vi "CloseIO.vi"   [LabVIEW 2012]
types:
  T1 = typedef "WPI_MotorControlDeviceRef.ctl" = cluster{"DeviceStatus":errorcluster, "Type":enum16{"PWM", "CAN"}, "PWM":cluster{"Digital Module":T2, "PWM Channel":T3, "DeadBand":T4}, "CAN":cluster{"Device Number":u8, "Control Mode":T5, "Semaphore":T6, "Max Vout":dbl}, "Invert":bool, "TransformRef":T7, "InvTransformRef":T7}
  T2 = typedef "FPGA_TypedefDigitalModule.ctl" = enum16{"Digital Module 1", "Digital Module 2"}
  T3 = typedef "FPGA_DIOPWMChannel.ctl" = enum8{"PWM 1", "PWM 2", "PWM 3", "PWM 4", "PWM 5", "PWM 6", "PWM 7", "PWM 8", "PWM 9", "PWM 10", "Invalid"}
  T4 = typedef "WPI_PWMDeadband.ctl" = cluster{"Name":string, "maxPositivePwm":i32, "minPositivePwm":i32, "centerPwm":i32, "maxNegativePwm":i32, "minNegativePwm":i32, "angularRange":u16}
  T5 = typedef "WPI_CANJaguar_ControlMode.ctl" = enum8{"Percent VBus", "Current", "Speed", "Position", "Voltage"}
  T6 = typedef "Semaphore RefNum" = refnum<k1>
  T7 = typedef "WPI_PWMTransform_ConPane.ctl" = refnum<vi>
  T8 = typedef "WPI_RobotDriveDevRef.ctl" = cluster{"DevStatus":errorcluster, "Motors[]":T1[], "Square Inputs":bool, "Max Output":dbl, "Isochronous":bool}
  T9 = typedef "WPI_DigitalInputDevRef.ctl" = cluster{"DevStatus":errorcluster, "DIO Channel":T10, "Digital Module":T2}
  T10 = typedef "FPGA_DIOChannel.ctl" = enum8{"DIO 1", "DIO 2", "DIO 3", "DIO 4", "DIO 5", "DIO 6", "DIO 7", "DIO 8", "DIO 9", "DIO 10", "DIO 11", "DIO 12", "DIO 13", "DIO 14", "Invalid"}
  T11 = typedef "WPI_CounterDevRef.ctl" = cluster{"DevStatus":errorcluster, "CntIndex":T12}
  T12 = typedef "FPGA_CounterCtrSystemIndex.ctl" = enum8{"Ctr 0", "Ctr 1", "Ctr 2", "Ctr 3", "Ctr 4", "Ctr 5", "Ctr 6", "Ctr 7", "Invalid"}
  T13 = typedef "WPI_EncoderDevRef.ctl" = cluster{"DevStatus":errorcluster, "EncoderIndex":T14, "CounterIndex":T12, "DistancePerCount":dbl, "Decoding Type":T15}
  T14 = typedef "FPGA_EncoderIdx.ctl" = enum8{"Enc 0", "Enc 1", "Enc 2", "Enc 3", "Invalid"}
  T15 = typedef "WPI_EncoderType.ctl" = enum16{"1x", "2x", "4x"}
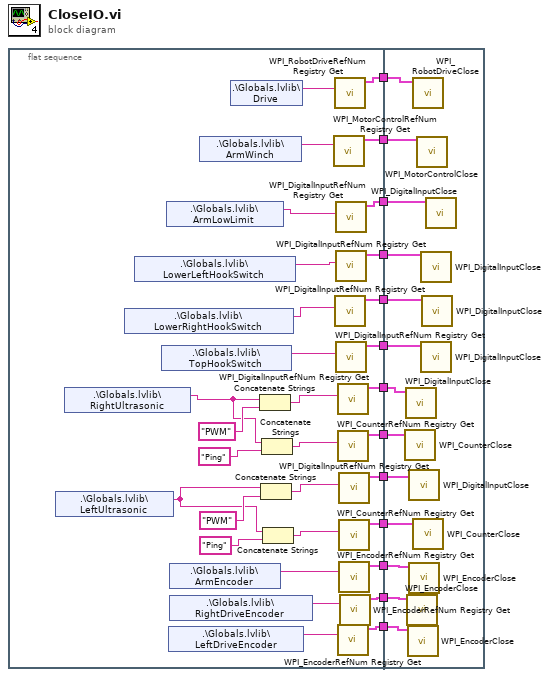
[diagram p0: block diagram]
diagram:
  n1 = flat-sequence {
    tunnel: [w43] -> w13
    tunnel: [w42] -> w12
    tunnel: [w27] -> w11
    tunnel: [w26] -> w10
    tunnel: [w25] -> w9
    tunnel: [w24] -> w8
    tunnel: [w23] -> w7
    tunnel: [w22] -> w6
    tunnel: [w21] -> w5
    tunnel: [w20] -> w4
    tunnel: [w18] -> w3
    tunnel: [w17] -> w2
    tunnel: [w14] -> w1
    tunnel: w13 -> [w58]
    tunnel: w12 -> [w57]
    tunnel: w11 -> [w56]
    tunnel: w10 -> [w55]
    tunnel: w9 -> [w54]
    tunnel: w8 -> [w53]
    tunnel: w7 -> [w52]
    tunnel: w6 -> [w51]
    tunnel: w5 -> [w50]
    tunnel: w4 -> [w49]
    tunnel: w3 -> [w48]
    tunnel: w2 -> [w47]
    tunnel: w1 -> [w46]
    frame #0 {
      n2 = shared-variable ".\\Globals.lvlib\\LeftUltrasonic"() -> (w29:string)  [unwired: 1 in, 1 out]
      n3 = shared-variable ".\\Globals.lvlib\\RightUltrasonic"() -> (w35:string)  [unwired: 1 in, 1 out]
      n4 = shared-variable ".\\Globals.lvlib\\LowerRightHookSwitch"() -> (w39:string)  [unwired: 1 in, 1 out]
      n5 = shared-variable ".\\Globals.lvlib\\LowerLeftHookSwitch"() -> (w40:string)  [unwired: 1 in, 1 out]
      n6 = shared-variable ".\\Globals.lvlib\\TopHookSwitch"() -> (w38:string)  [unwired: 1 in, 1 out]
      n7 = shared-variable ".\\Globals.lvlib\\ArmLowLimit"() -> (w41:string)  [unwired: 1 in, 1 out]
      n8 = shared-variable ".\\Globals.lvlib\\LeftDriveEncoder"() -> (w15:string)  [unwired: 1 in, 1 out]
      n9 = shared-variable ".\\Globals.lvlib\\ArmEncoder"() -> (w16:string)  [unwired: 1 in, 1 out]
      n10 = shared-variable ".\\Globals.lvlib\\RightDriveEncoder"() -> (w19:string)  [unwired: 1 in, 1 out]
      n11 = shared-variable ".\\Globals.lvlib\\ArmWinch"() -> (w44:string)  [unwired: 1 in, 1 out]
      n12 = shared-variable ".\\Globals.lvlib\\Drive"() -> (w45:string)  [unwired: 1 in, 1 out]
      n13 = Concatenate Strings(w35, "PWM") -> (w36:string)
      n14 = Concatenate Strings(w29, "PWM") -> (w31:string)
      n15 = Concatenate Strings(w35, "Ping") -> (w33:string)
      n16 = Concatenate Strings(w29, "Ping") -> (w32:string)
      n17 = call <vilib>:"WPI_MotorControlRefNum Registry Get.vi"("refnum name"=w44) -> ("MotorControlDevRef"=w42:T1)  [unwired: 9 in, 1 out]
      n18 = call <vilib>:"WPI_RobotDriveRefNum Registry Get.vi"("refnum name"=w45) -> ("RobotDriveDevRef"=w43:T8)  [unwired: 9 in, 1 out]
      n19 = call <vilib>:"WPI_DigitalInputRefNum Registry Get.vi"("refnum name"=w39) -> ("DigitalInputDevRef"=w24:T9)  [unwired: 9 in, 1 out]
      n20 = call <vilib>:"WPI_DigitalInputRefNum Registry Get.vi"("refnum name"=w41) -> ("DigitalInputDevRef"=w22:T9)  [unwired: 9 in, 1 out]
      n21 = call <vilib>:"WPI_DigitalInputRefNum Registry Get.vi"("refnum name"=w40) -> ("DigitalInputDevRef"=w23:T9)  [unwired: 9 in, 1 out]
      n22 = call <vilib>:"WPI_DigitalInputRefNum Registry Get.vi"("refnum name"=w38) -> ("DigitalInputDevRef"=w25:T9)  [unwired: 9 in, 1 out]
      n23 = call <vilib>:"WPI_DigitalInputRefNum Registry Get.vi"("refnum name"=w36) -> ("DigitalInputDevRef"=w26:T9)  [unwired: 9 in, 1 out]
      n24 = call <vilib>:"WPI_CounterRefNum Registry Get.vi"("refnum name"=w33) -> ("CounterDevRef"=w20:T11)  [unwired: 9 in, 1 out]
      n25 = call <vilib>:"WPI_EncoderRefNum Registry Get.vi"("refnum name"=w15) -> ("EncoderDevRef"=w14:T13)  [unwired: 9 in, 1 out]
      n26 = call <vilib>:"WPI_DigitalInputRefNum Registry Get.vi"("refnum name"=w31) -> ("DigitalInputDevRef"=w27:T9)  [unwired: 9 in, 1 out]
      n27 = call <vilib>:"WPI_CounterRefNum Registry Get.vi"("refnum name"=w32) -> ("CounterDevRef"=w21:T11)  [unwired: 9 in, 1 out]
      n28 = call <vilib>:"WPI_EncoderRefNum Registry Get.vi"("refnum name"=w16) -> ("EncoderDevRef"=w17:T13)  [unwired: 9 in, 1 out]
      n29 = call <vilib>:"WPI_EncoderRefNum Registry Get.vi"("refnum name"=w19) -> ("EncoderDevRef"=w18:T13)  [unwired: 9 in, 1 out]
    }
    frame #1 {
      n30 = call <vilib>:"WPI_CounterClose.vi"("CounterDevRef"=w49) -> ()  [unwired: 10 in, 1 out]
      n31 = call <vilib>:"WPI_DigitalInputClose.vi"("DigitalInputDevRef"=w55) -> ()  [unwired: 10 in, 1 out]
      n32 = call <vilib>:"WPI_EncoderClose.vi"("EncoderDevRef"=w48) -> ()  [unwired: 10 in, 1 out]
      n33 = call <vilib>:"WPI_EncoderClose.vi"("EncoderDevRef"=w46) -> ()  [unwired: 10 in, 1 out]
      n34 = call <vilib>:"WPI_DigitalInputClose.vi"("DigitalInputDevRef"=w56) -> ()  [unwired: 10 in, 1 out]
      n35 = call <vilib>:"WPI_EncoderClose.vi"("EncoderDevRef"=w47) -> ()  [unwired: 10 in, 1 out]
      n36 = call <vilib>:"WPI_RobotDriveClose.vi"("RobotDriveDevRef"=w58) -> ()  [unwired: 10 in, 1 out]
      n37 = call <vilib>:"WPI_CounterClose.vi"("CounterDevRef"=w50) -> ()  [unwired: 10 in, 1 out]
      n38 = call <vilib>:"WPI_MotorControlClose.vi"("MotorControlDevRef"=w57) -> ()  [unwired: 10 in, 1 out]
      n39 = call <vilib>:"WPI_DigitalInputClose.vi"("DigitalInputDevRef"=w52) -> ()  [unwired: 10 in, 1 out]
      n40 = call <vilib>:"WPI_DigitalInputClose.vi"("DigitalInputDevRef"=w54) -> ()  [unwired: 10 in, 1 out]
      n41 = call <vilib>:"WPI_DigitalInputClose.vi"("DigitalInputDevRef"=w53) -> ()  [unwired: 10 in, 1 out]
      n42 = call <vilib>:"WPI_DigitalInputClose.vi"("DigitalInputDevRef"=w51) -> ()  [unwired: 10 in, 1 out]
    }
  }
